vi "Daisy Chain 1.vi"   [LabVIEW 2016, in "Moving Motor.lvrbt"]
uses:
  Moving Motor.lvrbt
  <vilib>/NXT/Block Support/NXT_OutputPort.ctl
  <vilib>/NXT/NXTIO Xnodes/NXTIONodeSubVIs/NXTMoveMotors.vi
  <vilib>/NXT/Subs/LVHSConnector.ctl
  <vilib>/NXT/NXTIO Xnodes/AddressXNode/NXTIOAddress.xnode
  <vilib>/NXT/NXTIO Xnodes/NXTIOXNode/NXTIO.xnode
  <vilib>/NXT/LegoClasses/BrickReference/BrickReference.lvclass
types:
  T1 = typedef "NXT_OutputPort.ctl" = u8
  T2 = typedef "LVHSConnector.ctl" = refnum<class "BrickReference.lvclass">
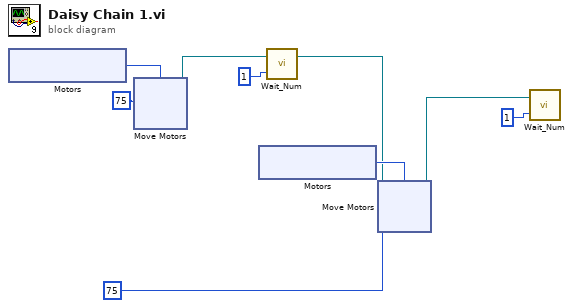
[diagram p0: block diagram]
diagram:
  n1 = xnode "Motors"() -> ("Motor"=w9:T1)
  n2 = xnode "Move Motors"("Power/Speed 1"=75, "Motors"=w9) -> ("NXT/EV3"=w6:T2)  [unwired: 1 in]
  n3 = xnode "Motors"() -> ("Motor"=w8:T1)
  n4 = call <vilib>:"Wait_Num.vi"("Time (1 sec)"=1, "NXT/EV3"=w6) -> ("NXT/EV3"=w5:T2)  [unwired: 2 in]
  n5 = xnode "Move Motors"("Power/Speed 1"=75, "Motors"=w8, "NXT/EV3"=w5) -> ("NXT/EV3"=w1:T2)
  n6 = call <vilib>:"Wait_Num.vi"("Time (1 sec)"=1, "NXT/EV3"=w1) -> ()  [unwired: 2 in, 1 out]
